vi "Webcam grab example.vi"() -> ()   [LabVIEW 2013]
doc: "The Low-Level Grab Raw Data VI acquires images continuously using low-level acquisition VIs. This VI demonstrates how to acquire raw data from the camera. A grab is appropriate for high-speed applications in which you need to process only one image at a time."
uses:
  <vilib>/vision/driver/IMAQdx.llb/IMAQdx Acquisition Mode.ctl
  <vilib>/vision/driver/IMAQdx.llb/IMAQdx Buffer Number Mode.ctl
  <vilib>/vision/driver/NI_Vision_Acquisition_Software.lvlib
  <resource>/objmgr/imaqdx.rc
panel:
  out "Tube Position":i16[](graph)
  in  "index":i32
  out "Tube ROI":i16[][](graph)
  in  "bird index":i32=35
  out "Tube":i16[][](graph)
  out "y value":i32(slide) scale=0.0..160.0
  out "Bird Position":i16[](graph)
  out "RED ROI":i16[][](graph)
  out "Bird":i16[][](graph)
  out "Red":i16[][](graph)
  out "Green":i16[][](graph)
  out "Blue":i16[][](graph)
  in  "Camera Name":refnum<k21> caption="IMAQdx Session"
  out "Buffer Number":u32
  in  "Stop":bool
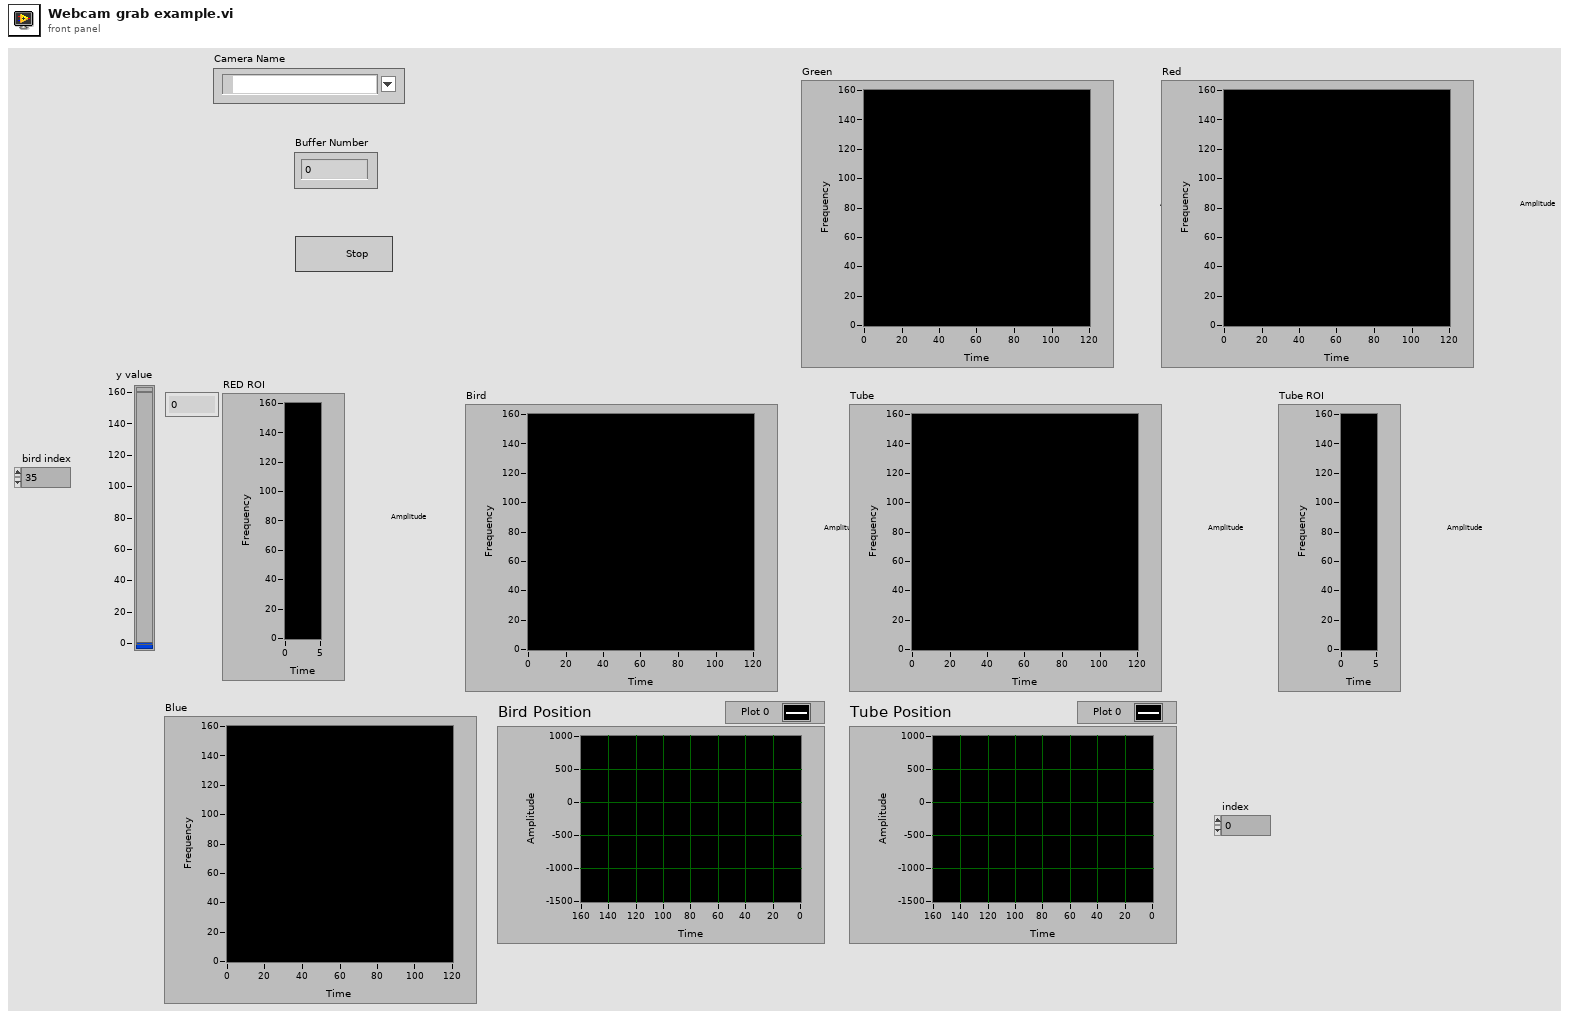
[diagram p1: front panel]
types:
  T1 = typedef "NI_Vision_Acquisition_Software.lvlib/IMAQdx Acquisition Mode.ctl" = enum32{"One Shot", "Continuous"}
  T2 = typedef "IMAQdx.ctl" = refnum<k21>
  T3 = typedef "NI_Vision_Acquisition_Software.lvlib/IMAQdx Buffer Number Mode.ctl" = enum32{"Next", "Last", "Buffer Number"}
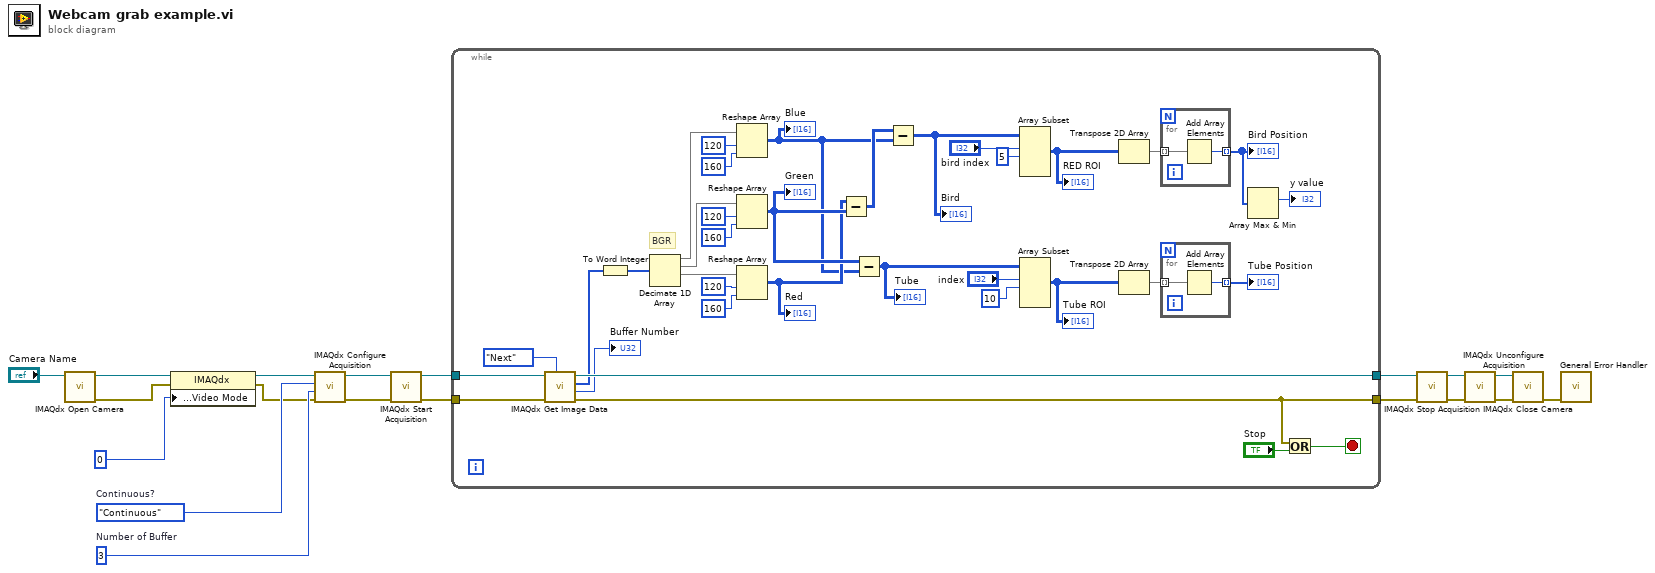
[diagram p0: block diagram]
diagram:
  w8 = IMAQdx_Acquisition_Mode."Continuous"  # Continuous?
  w18 = u32 3  # Number of Buffer
  n1 = call <vilib>:"IMAQdx Open Camera.vi"("Session In"="Camera Name") -> ("error out"=w2:errorcluster, "Session Out"=w4:T2)  [unwired: 2 in, 7 out]
  n2 = property class="IMAQdx"(reference=w4, error in=w2, "Acquisition Attributes:Video Mode"=u32 0 ("VideoMode")) -> (reference out=w3:T2, error out=w1:errorcluster)
  n3 = call <vilib>:"IMAQdx Configure Acquisition.vi"("error in"=w1, "Number of Buffers"=w18, "Continuous?"=w8, "Session In"=w3) -> ("error out"=w5:errorcluster, "Session Out"=w6:T2)  [unwired: 6 out]
  n4 = call <vilib>:"IMAQdx Start Acquisition.vi"("error in"=w5, "Session In"=w6) -> ("error out"=w17:errorcluster, "Session Out"=w16:T2)  [unwired: 8 out]
  n5 = while {
    tunnel: [w51] -> w14
    tunnel: w17 -> [w52]
    tunnel: w16 -> [w53]
    tunnel: [w48] -> w15
    stop <- w55 stop-if-true
    # "BGR"
    n6 = call <vilib>:"IMAQdx Get Image Data.vi"("Buffer Number Mode (Next)"=IMAQdx_Buffer_Number_Mode."Next", "error in"=w52, "Session In"=w53) -> ("error out"=w48:errorcluster, "Buffer Number Out"=→"Buffer Number":u32, "Image Data Array"=w44:u8[], "Session Out"=w51:T2)  [unwired: 1 in, 4 out]
    n7 = To Word Integer(number=w44) -> (16bit integer=w43:i16[])
    n8 = Decimate 1D Array(w43) -> (w45:i16[], w37:i16[], w38:i16[])  [unwired: 1 out]
    n9 = Reshape Array(w45, 120 ("index"), u8 160 ("new element/subarray")) -> (w26:i16[][])
    "Blue" <- w26
    n10 = Reshape Array(w37, 120 ("index"), u8 160 ("new element/subarray")) -> (w28:i16[][])
    "Green" <- w28
    n11 = Reshape Array(w38, 120 ("index"), u8 160 ("new element/subarray")) -> (w27:i16[][])
    "Red" <- w27
    n12 = Subtract(x=w27, y=w28) -> (x-y=w36:i16[][])
    n13 = Subtract(x=w28, y=w26) -> (x-y=w25:i16[][])
    "Tube" <- w25
    n14 = Subtract(x=w36, y=w26) -> (x-y=w35:i16[][])
    "Bird" <- w35
    n15 = Array Subset(array=w35, index (row)="bird index", length (row)=5 ("length")) -> (w31:i16[][])  [unwired: 2 in]
    "RED ROI" <- w31
    n16 = Array Subset(array=w25, index (row)="index", length (row)=10 ("length")) -> (w21:i16[][])  [unwired: 2 in]
    "Tube ROI" <- w21
    n17 = Transpose 2D Array(2D array=w31) -> (transposed array=w32:i16[][])
    n18 = Transpose 2D Array(2D array=w21) -> (transposed array=w22:i16[][])
    n19 = for {
      tunnel: w32 -> [w59] mode=indexing
      tunnel: [w58] -> w30 mode=indexing
      n20 = Add Array Elements(numeric array=w59) -> (sum=w58:i16)
    }
    "Bird Position" <- w30
    n21 = for {
      tunnel: w22 -> [w57] mode=indexing
      tunnel: [w56] -> w23 mode=indexing
      n22 = Add Array Elements(numeric array=w57) -> (sum=w56:i16)
    }
    "Tube Position" <- w23
    n23 = Array Max & Min(array=w30) -> (max index (indices)=→"y value":i32)  [unwired: 3 out]
    n24 = Or(x=w48, y="Stop") -> (x .or. y?=w55:bool)
  }
  n25 = call <vilib>:"IMAQdx Stop Acquisition.vi"("error in"=w15, "Session In"=w14) -> ("error out"=w13:errorcluster, "Session Out"=w12:T2)  [unwired: 8 out]
  n26 = call <vilib>:"IMAQdx Unconfigure Acquisition.vi"("error in"=w13, "Session In"=w12) -> ("error out"=w10:errorcluster, "Session Out"=w11:T2)  [unwired: 8 out]
  n27 = call <vilib>:"IMAQdx Close Camera.vi"("error in"=w10, "Session In"=w11) -> ("error out"=w19:errorcluster)  [unwired: 9 out]
  n28 = call <vilib>:"General Error Handler.vi"("error in (no error)"=w19) -> ()  [unwired: 1 in, 14 out]
